vi "Configure Multi Eval Meas Modulation EVM Window Length Selected BW.vi"(6 "SCS 120kHz (1)":i32=1, 7 "SCS 60kHz (1)":i32=1, 8 "error in (no error)":errorcluster, 9 "Bandwidth (50 MHz)":T1 items=["50 MHz", "100 MHz", "200 MHz", "400 MHz"], 10 "Instance (1)":T2=1, 11 "VISA resource name":refnum<visa-resource-name>) -> (0 "error out":errorcluster, 3 "VISA resource name out":refnum<visa-resource-name>)   [LabVIEW 2020, in "Rohde&Schwarz CMXP NR FR2 Measurement.lvlib"]
doc: "Specifies the EVM window length in samples for a selected channel bandwidth, depending on the SC spacing.\n\nAttribute:\nRSCMXPNRFR2M_ATTR_MULTI_EVAL_MEASUREMENT_MODULATION_EVM_WINDOW_LENGTH_SELECTED_BW\n\nRemote-control command:\nCONFigure:NRMMw:MEAS<i>:MEValuation:MODulation:EWLength:CBANdwidth<bw>"
uses:
  <instrlib>/Rohde&Schwarz CMXP NR FR2 Measurement/Rohde&Schwarz CMXP NR FR2 Measurement.lvlib
  <instrlib>/Rohde&Schwarz CMXP NR FR2 Measurement/Private/_Instance.ctl
  <instrlib>/Rohde&Schwarz CMXP NR FR2 Measurement/Private/_Bandwidth.ctl
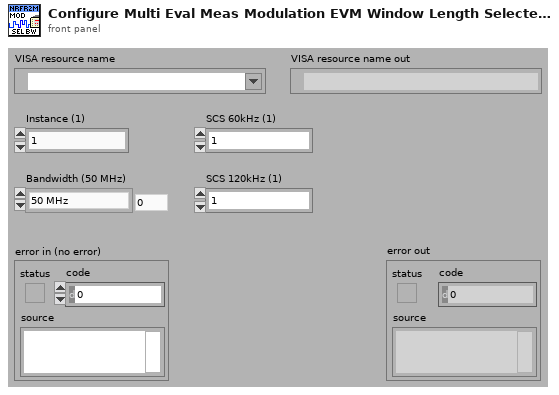
[diagram p1: front panel]
types:
  T1 = typedef "Rohde&Schwarz CMXP NR FR2 Measurement.lvlib/_Bandwidth.ctl" = i32
  T2 = typedef "Rohde&Schwarz CMXP NR FR2 Measurement.lvlib/_Instance.ctl" = i32
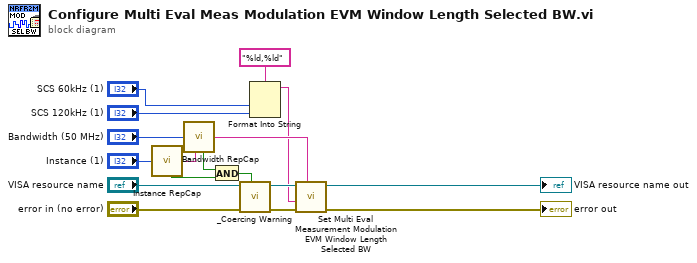
[diagram p0: block diagram]
diagram:
  n1 = call <instrlib>:"Instance RepCap.vi"("Instance In"="Instance (1)") -> ("In Range?"=w14:bool, "RepCap Identifier Out"=w2:string)  [unwired: 1 in]
  n2 = call <instrlib>:"Bandwidth RepCap.vi"("Bandwidth In"="Bandwidth (50 MHz)", "RepCap String In (\"\")"=w2) -> ("In Range?"=w13:bool, "RepCap Identifier Out"=w9:string)
  n3 = And(x=w13, y=w14) -> (x .and. y?=w4:bool)
  n4 = call <instrlib>:"_Coercing Warning.vi"("In Range?"=w4, "error in (no error)"="error in (no error)", "VISA resource name"="VISA resource name") -> ("error out"=w7:errorcluster, "VISA resource name out"=w8:refnum<visa-resource-name>)  [unwired: 7 in]
  n5 = Format Into String(format string="%ld,%ld", "SCS 60kHz (1)", "SCS 120kHz (1)") -> (resulting string=w1:string)  [unwired: 2 in, 1 out]
  n6 = call "Set Multi Eval Measurement Modulation EVM Window Length Selected BW"("Repeated Capabilities"=w9, "error in (no error)"=w7, "Multi Eval Measurement Modulation EVM Window Length Selected BW ()"=w1, "instrument handle"=w8) -> ("error out"=→"error out":errorcluster, "instrument handle out"=→"VISA resource name out":refnum<visa-resource-name>)  [unwired: 6 in]
